vi "HarvesterManual.vi"() -> ()   [LabVIEW 2013]
panel:
  out "Power":dbl
  in  "HarvOutPos":dbl=5.0
  in  "HarvInPos":dbl
  in  "HarvPot":dbl
  in  "HarvButtonOut":bool
  in  "HarvButtonIn":bool
  in  "HarvLimitIn":bool
  in  "HarvLimitOut":bool
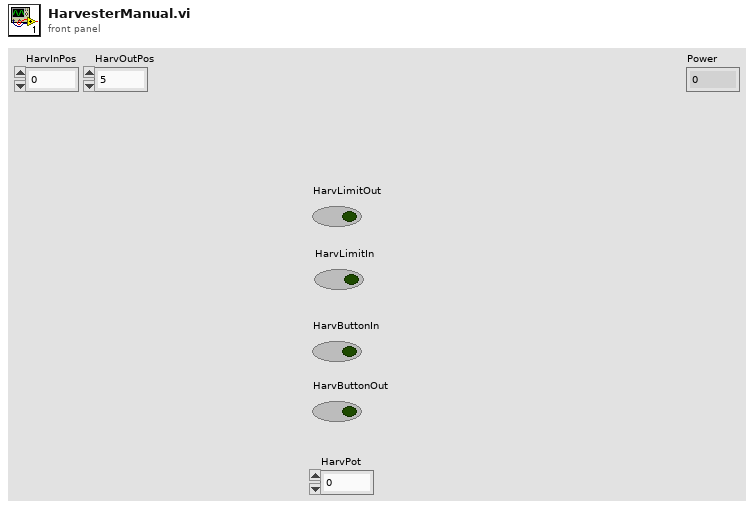
[diagram p1: front panel]
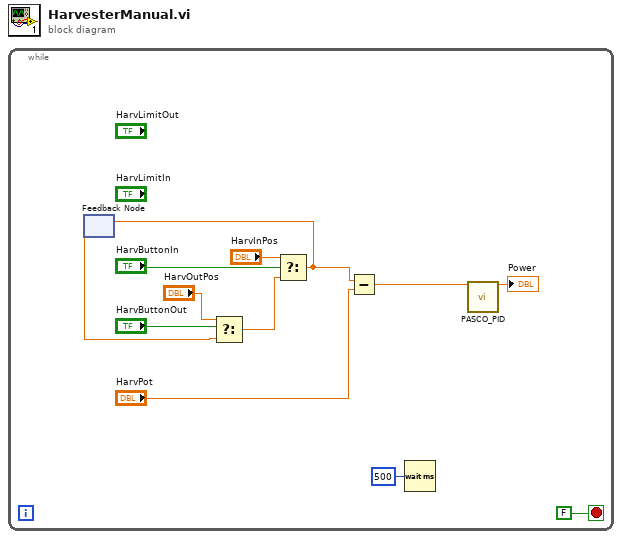
[diagram p0: block diagram]
diagram:
  n1 = while {
    stop <- FALSE stop-if-true
    n2 = feedback #1() -> (w9:dbl)  [unwired: 1 in]
    n3 = Select(t="HarvOutPos", s="HarvButtonOut", f=w9) -> (s? t:f=w10:dbl)
    n4 = Select(t="HarvInPos", s="HarvButtonIn", f=w10) -> (s? t:f=w6:dbl)
    n5 = feedback-in #1(w6) -> ()
    n6 = Subtract(x=w6, y="HarvPot") -> (x-y=w4:dbl)
    n7 = Wait (ms)(milliseconds to wait=u32 500) -> ()  [unwired: 1 out]
    n8 = call "PASCO_PID.vi"("Delta"=w4) -> ("Output"=→"Power":dbl)  [unwired: 13 in, 1 out]
  }
